vi "MenuBuild.vi"(0 "MenuCol in":refnum<class "MenuCol.lvclass">, 1 "row type":T2, 3 "Clipboard":refnum<vi>, 5 "MenuRef In":refnum<k9>, 7 "Click Position":T1, 9 "Table CtlRef In":refnum<vi>, 11 "error in (no error)":errorcluster, 12 "withinSelection?":bool=TRUE, 14 "Button\n(Mouse Down?)":u16) -> (4 "MenuCol out":refnum<class "MenuCol.lvclass">, 6 "MenuRef Out":refnum<k9>, 10 "Table CtlRef Out":refnum<vi>, 15 "error out":errorcluster)   [LabVIEW 2013, in "MenuCol.lvclass"]
doc: "Build shortcut (right-click) menu items for all columns in general. This VI is read-only w.r.t column data."
uses:
  MenuCol.lvclass
  TypeDefs/RowType.ctl
  <vilib>/Utility/miscctls.llb/LVRowAndColumnTypeDef.ctl
  Column/Column.lvclass
panel:
  # "needed when providing multiple\nshortcut menus based on which\nmouse button clicked.\ne.g. LMenuCol override of\nMenuBuild method."
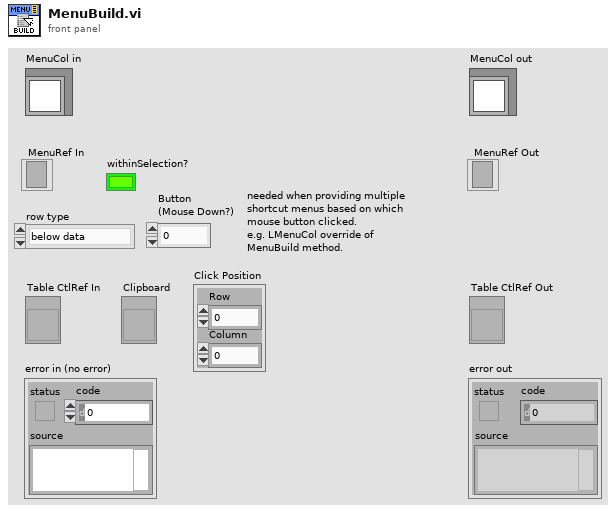
[diagram p1: front panel]
types:
  T1 = typedef "LVRowAndColumnTypeDef.ctl" = cluster{"Row":i32, "Column":i32}
  T2 = typedef "RowType.ctl" = enum16{"below data", "within data", "column header", "first row"}
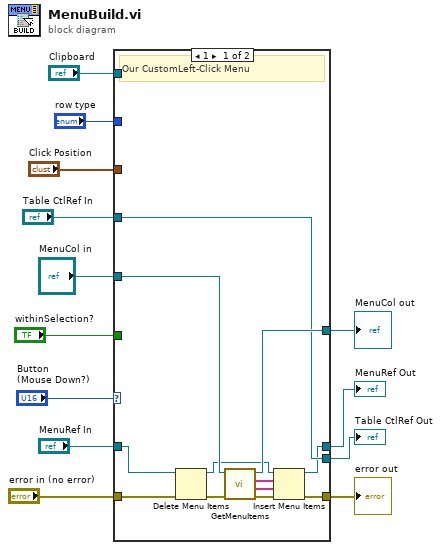
[diagram p0: block diagram]
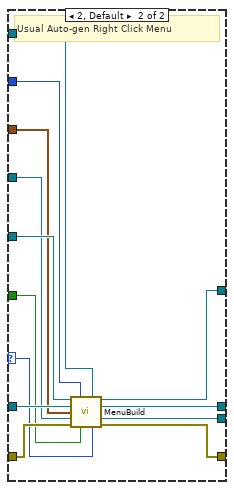
[diagram p2: hidden frame]
diagram:
  n1 = case shown="1" "Button\n(Mouse Down?)" {
    selector: "Button\n(Mouse Down?)" -> [_ w26]
    tunnel: "MenuCol in" -> [w25 w38]
    tunnel: "row type" -> [_ w37]
    tunnel: "Clipboard" -> [_ w36]
    tunnel: [w24 w35] -> w10
    tunnel: "MenuRef In" -> [w22 w34]
    tunnel: [w14 w33] -> w8
    tunnel: "Click Position" -> [_ w32]
    tunnel: "Table CtlRef In" -> [w23 w31]
    tunnel: [w23 w30] -> w5
    tunnel: "error in (no error)" -> [w21 w29]
    tunnel: "withinSelection?" -> [_ w28]
    tunnel: [w19 w27] -> w2
    frame 1 {
      # "Our CustomLeft-Click Menu"
      n2 = Delete Menu Items(6:w21, 9:w22) -> (0:w20:errorcluster, 3:w15:refnum<k9>)  [unwired: 2 in]
      n3 = call-dynamic "GetMenuItems.vi"("error in (no error)"=w20, "MenuCol in"=w25) -> ("error out"=w18:errorcluster, "MenuTags"=w17:string[], "MenuLabels"=w16:string[], "MenuCol out"=w24:refnum<class "MenuCol.lvclass">)  [unwired: 6 in]
      n4 = Insert Menu Items(6:w18, 7:w17, 8:w16, 9:w15) -> (0:w19:errorcluster, 3:w14:refnum<k9>)  [unwired: 2 in, 1 out]
    }
    frame 2, Default {
      # "Usual Auto-gen Right Click Menu"
      n5 = call-parent "MenuBuild.vi"("Column in"=w38, "row type"=w37, "Clipboard"=w36, "MenuRef In"=w34, "Click Position"=w32, "Table CtlRef In"=w31, "error in (no error)"=w29, "withinSelection?"=w28, "Button\n(Mouse Down?)"=w26) -> ("Column out"=w35:refnum<class "MenuCol.lvclass">, "MenuRef Out"=w33:refnum<k9>, "Table CtlRef Out"=w30:refnum<vi>, "error out"=w27:errorcluster)  [unwired: 3 in]
    }
  }
  "error out" <- w2
  "MenuCol out" <- w10
  "MenuRef Out" <- w8
  "Table CtlRef Out" <- w5
